vi "Test One to Many Relation.vi"() -> ()   [LabVIEW 2020, in "Test.lvlib"]
uses:
  Test.lvlib
  Conditum SQLite/SQLite/SQLite.lvclass
  User/User.lvclass
  <vilib>/IlluminatedG/IG Conditum Base/Conditum/Entity Manager/Entity Manager.lvclass
  <vilib>/IlluminatedG/IG Conditum Base/Conditum/Entity ID.ctl
  <vilib>/IlluminatedG/IG Conditum Base/Conditum/Conditum.lvlib
  C:/Program Files (x86)/National Instruments/LabVIEW 2020/vi.lib/IlluminatedG/IG Conditum Base/Conditum/Database Platform/Database Platform.lvclass
  C:/dev/lv20CE/lv-conditum-sqlite/Conditum SQLite/SQLite/SQLite.lvclass
  C:/Program Files (x86)/National Instruments/LabVIEW 2020/vi.lib/IlluminatedG/IG Conditum Base/Conditum/Entity/Entity.lvclass
  C:/dev/lv20CE/lv-conditum-sqlite/Test/User/User.lvclass
panel:
  in  "DB Path":path=path "C:/dev/lv20CE/lv-conditum-sqlite/Test/test.db"
  in  "New Email":string
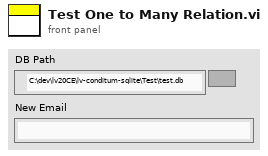
[diagram p1: front panel]
types:
  T1 = typedef "Conditum.lvlib/Entity ID.ctl" = i64
  T2 = typedef "Test.lvlib/User.lvclass/Values.ctl" = cluster{"Username":string, "Password":string, "Joined":timestamp, "Last Activity":timestamp, "Activated":bool, "Email":string, "Score":i64}
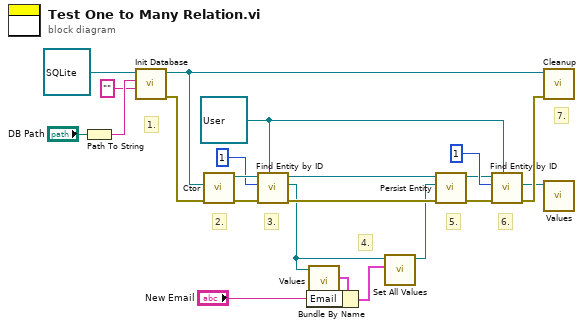
[diagram p0: block diagram]
diagram:
  w1 = refnum<class "User.lvclass"> refnum ("Test.lvlib:User.lvclass")
  # "7."
  # "6."
  # "5."
  # "4."
  # "3."
  # "2."
  # "1."
  n1 = Path To String(path="DB Path") -> (string=w19:string)
  n2 = call-dynamic "Init Database.vi"("Database"="", "Resource"=w19, "Database in"=refnum<class "SQLite.lvclass"> refnum) -> ("error out"=w16:errorcluster, "Database out"=w15:refnum<class "SQLite.lvclass">)  [unwired: 7 in]
  n3 = call <vilib>:"Ctor.vi"("error in (no error)"=w16, "Database"=w15) -> ("error out"=w21:errorcluster, "Entity Manager out"=w14:refnum<class "Entity Manager.lvclass">)  [unwired: 8 in]
  n4 = call <vilib>:"Find Entity by ID.vi"("Entity Type"=w1, "error in (no error)"=w21, "Entity ID"=T1 1, "Entity Manager in"=w14) -> ("error out"=w22:errorcluster, "Entity"=w10:refnum<class "User.lvclass">, "Entity Manager out"=w8:refnum<class "Entity Manager.lvclass">)  [unwired: 5 in]
  n5 = call "Values.vi"("User in"=w10) -> ("Values"=w12:T2)  [unwired: 10 in]
  n6 = Bundle By Name(cluster=w12, "Email"="New Email") -> (w9:T2)
  n7 = call "Set All Values.vi"("Values"=w9, "User in"=w10) -> ("User out"=w7:refnum<class "User.lvclass">)  [unwired: 8 in, 1 out]
  n8 = call <vilib>:"Persist Entity.vi"("error in (no error)"=w22, "Conditum:Entity"=w7, "Entity Manager in"=w8) -> ("error out"=w4:errorcluster, "Entity Manager out"=w5:refnum<class "Entity Manager.lvclass">)  [unwired: 7 in]
  n9 = call <vilib>:"Find Entity by ID.vi"("Entity Type"=w1, "error in (no error)"=w4, "Entity ID"=T1 1, "Entity Manager in"=w5) -> ("error out"=w3:errorcluster, "Entity"=w2:refnum<class "User.lvclass">)  [unwired: 5 in, 1 out]
  n10 = call-dynamic "Cleanup.vi"("error in (no error)"=w3, "SQLite in"=w15) -> ()  [unwired: 9 in, 1 out]
  n11 = call "Values.vi"("User in"=w2) -> ()  [unwired: 10 in, 1 out]
